vi "create RCVR files.vi"(11 "Name of RCVR 1":string="RCVR 1" caption="Name of RCVR") -> (1 "error out":errorcluster, 2 "refnum out":refnum<file>, 3 "Name of file out":string)   [LabVIEW 2011]
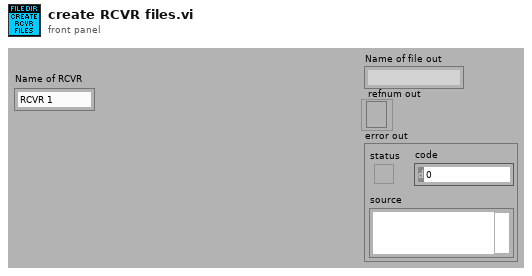
[diagram p1: front panel]
types:
  T1 = cluster{"Number of hours To Collect before starting new file ":u16, "Base File Path":path, "Update setup":bool, "Shutdown software":bool, "Time between samples (seconds)":u32}
  T2 = enum16{"open", "replace", "create", "open or create", "replace or create", "replace or create with confirmation"}
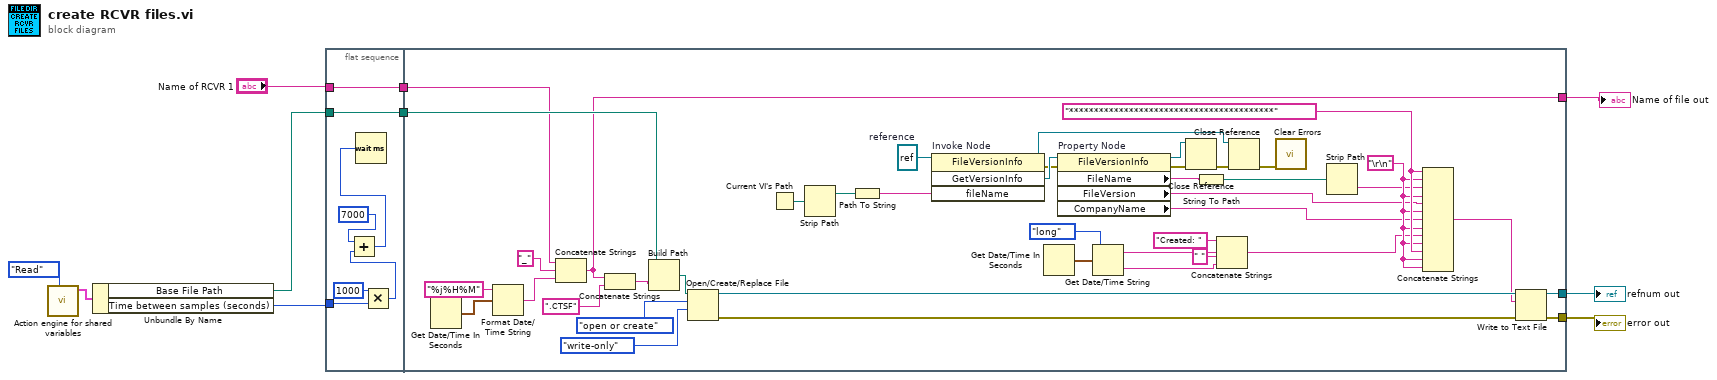
[diagram p0: block diagram]
diagram:
  n1 = call "Action engine for shared variables.vi"("read/write"=enum16{"Read", "Write"}."Read") -> ("func global variables read"=w3:T1)  [unwired: 9 in, 1 out]
  n2 = Unbundle By Name(w3) -> ("Base File Path"=w2:path, "Time between samples (seconds)"=w1:u32)
  n3 = flat-sequence {
    tunnel: w2 -> [w17]
    tunnel: [w17] -> w10
    tunnel: "Name of RCVR 1" -> [w12]
    tunnel: [w12] -> w8
    tunnel: w1 -> [w11]
    tunnel: [w45] -> w6
    tunnel: [w44] -> w5
    tunnel: w10 -> [w52]
    tunnel: [w49] -> w7
    tunnel: w8 -> [w48]
    frame #0 {
      n4 = Multiply(x=u32 1000, y=w11) -> (x*y=w15:u32)
      n5 = Add(x=u32 7000 ("milliseconds to wait"), y=w15) -> (x+y=w13:u32)
      n6 = Wait (ms)(milliseconds to wait=w13) -> ()  [unwired: 1 out]
    }
    frame #1 {
      w32 = refnum<k24> refnum  # reference
      w42 = "\r\n"
      w43 = "*****************************************" ("string")
      n7 = Get Date/Time In Seconds() -> (seconds since 1Jan1904=w54:timestamp)
      n8 = Format Date/Time String(time format string (%c)="%j%H%M", seconds (now)=w54) -> (date/time string=w55:string)  [unwired: 1 in]
      n9 = Concatenate Strings(w48, "_" ("string"), w55) -> (w49:string)
      n10 = Concatenate Strings(w49, ".CTSF" ("string")) -> (w50:string)
      n11 = Build Path(base path=w52, name or relative path=w50) -> (appended path=w57:path)
      n12 = Open/Create/Replace File(file path (use dialog)=w57, operation (0:open)=T2."open or create", access (0:read/write)=enum16{"read/write", "read-only", "write-only"}."write-only") -> (refnum out=w47:refnum<file>, error out=w46:errorcluster)  [unwired: 3 in, 1 out]
      n13 = Current VI's Path() -> (path=w31:path)
      n14 = Strip Path(path=w31) -> (stripped path=w30:path)  [unwired: 1 out]
      n15 = Path To String(path=w30) -> (string=w29:string)
      n16 = invoke on="Invoke Node" class="FileVersionInfo" method="GetVersionInfo"(reference=w32, "fileName"=w29) -> (reference out=w23:refnum<k24>, error out=w27:errorcluster, "GetVersionInfo"=w28:refnum<k24>)  [unwired: 2 in, 1 out]
      n17 = Get Date/Time In Seconds() -> (seconds since 1Jan1904=w35:timestamp)
      n18 = property on="Property Node" class="FileVersionInfo"(reference=w28, error in=w27) -> (reference out=w26:refnum<k24>, error out=w25:errorcluster, "FileName"=w20:string, "FileVersion"=w22:string, "CompanyName"=w21:string)
      n19 = Get Date/Time String(date format (0)=enum16{"short", "long", "abbreviated"}."long", seconds (now)=w35) -> (date string=w38:string, time string=w40:string)  [unwired: 1 in]
      n20 = Close Reference(reference=w26, error in (no error)=w25) -> (error out=w24:errorcluster)
      n21 = String To Path(string=w20) -> (path=w19:path)
      n22 = Concatenate Strings("Created: " ("string"), w38, " " ("string"), w40) -> (w41:string)
      n23 = Close Reference(reference=w23, error in (no error)=w24) -> (error out=w33:errorcluster)
      n24 = call <vilib>:"Clear Errors.vi"("error in (no error)"=w33) -> ()  [unwired: 6 in, 1 out]
      n25 = Strip Path(path=w19) -> (name=w18:string)  [unwired: 1 out]
      n26 = Concatenate Strings(w43, w42, w18, w42, w22, w42, w21, w42, w41, w42, w43, w42, w42) -> (w34:string)
      n27 = Write to Text File(file (use dialog)=w47, text=w34, error in=w46) -> (refnum out=w45:refnum<file>, error out=w44:errorcluster)  [unwired: 1 in, 1 out]
    }
  }
  "Name of file out" <- w7
  "refnum out" <- w6
  "error out" <- w5
